vi "Dequeue Element.vi"(6 "timeout in ms (-1)":i32=-1, 8 "error in (no error)":errorcluster, 11 "LVQueue Sink in":refnum<class "LVQueue Sink.lvclass">) -> (0 "error out":errorcluster, 2 "Log Packet":T1, 3 "LVQueue Sink out":refnum<class "LVQueue Sink.lvclass">, 4 "Timed Out?":bool)   [LabVIEW 2020, in "MVA Framework.lvlib" / "LVQueue Sink.lvclass"]
uses:
  LVQueue Sink.lvclass
  Composed Log/Types/Log Packet.ctl
  Composed Log/Types/Log Level.ctl
  LVQueue Sink.lvclass/LVQueue Sink.ctl
  Composed Log/Composed Log.lvlib
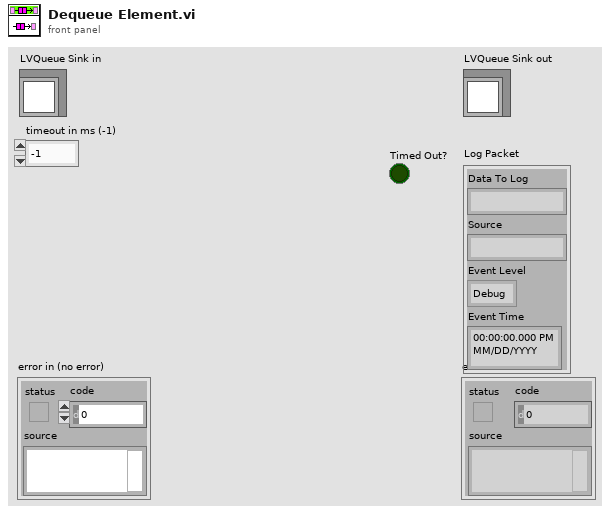
[diagram p1: front panel]
types:
  T1 = typedef "MVA Framework.lvlib/Composed Log.lvlib/Log Packet.ctl" = cluster{"Data To Log":string, "Source":string, "Event Level":T2, "Event Time":timestamp}
  T2 = typedef "MVA Framework.lvlib/Composed Log.lvlib/Log Level.ctl" = enum16{"Debug", "Info", "Warning", "Error", "Critical"}
  T3 = typedef "Composed Log.lvlib/Application Logger.lvclass/Log Packet.ctl" = cluster{"Data To Log":string, "Source":string, "Event Level":T4, "Event Time":timestamp}
  T4 = typedef "Composed Log.lvlib/Log Sink.lvclass/Log Level.ctl" = enum16{"Debug", "Info", "Warning", "Error", "Critical"}
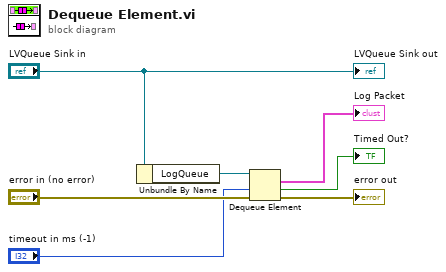
[diagram p0: block diagram]
diagram:
  n1 = Unbundle By Name("LVQueue Sink in") -> ("LogQueue"=w3:refnum<queue>)
  n2 = Dequeue Element(queue=w3, timeout in ms (-1)="timeout in ms (-1)", error in (no error)="error in (no error)") -> (element=→"Log Packet":T3, timed out?=→"Timed Out?":bool, error out=→"error out":errorcluster)  [unwired: 1 out]
  "LVQueue Sink out" <- "LVQueue Sink in"
